vi "Update Task Infos.vi"(8 "error in (no error)":errorcluster, 10 "Task":i32, 11 "Task Setting Editor in":refnum<class "Task Setting Editor.lvclass">) -> (0 "error out":errorcluster, 3 "Task Setting Editor out":refnum<class "Task Setting Editor.lvclass">)   [LabVIEW 2017, in "Task Setting Editor.lvlib" / "Task Setting Editor.lvclass"]
uses:
  Task Setting Editor.lvclass
  Task Setting Editor.lvclass/Task Setting Editor.ctl
  Classes/Task Interface/Task/Task.lvclass/Task.ctl
  Classes/Task Interface/Task/Get Name.vi
  Classes/Task Interface/Task/Get Target.vi
  Classes/Task Interface/Task/Read BuildSpec Type.vi
  Classes/Task Interface/Task/Get BuildSpec Name.vi
  Classes/Task Interface/Task/Get ProjectPath.vi
  Classes/Task Interface/Task/Read Worker.vi
  Classes/Task Interface/Task/Read Display Name.vi
  Classes/Task Interface/Task/Get Status String.vi
  Classes/Task Interface/Task/Get ProjectName.vi
  Classes/Task Interface/Task/Task.lvclass
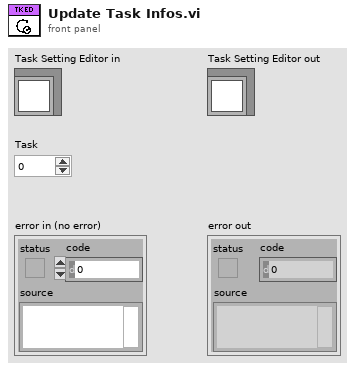
[diagram p1: front panel]
types:
  T1 = cluster{"Display Name":refnum<vi>, "Worker":refnum<vi>}
  T2 = cluster{"Name":refnum<vi>, "ProjectName":refnum<vi>, "Target":refnum<vi>, "BuildSpec Type":refnum<vi>, "BuildSpec Name":refnum<vi>, "ProjectPath":refnum<vi>, "Status string":refnum<vi>}
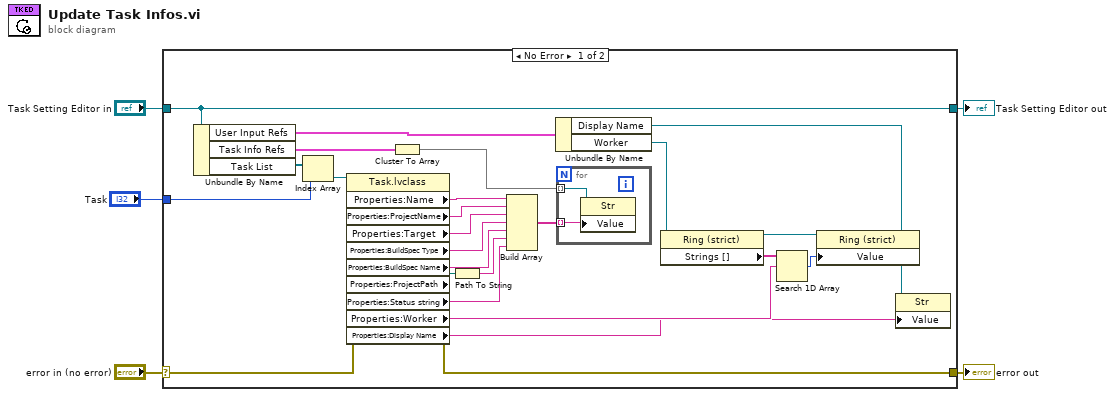
[diagram p0: block diagram]
diagram:
  n1 = case shown="No Error" "error in (no error)" {
    selector: "error in (no error)" -> [w27 w34]
    tunnel: [w26 w34] -> w4
    tunnel: [w30 w33] -> w2
    tunnel: "Task Setting Editor in" -> [w30 w33]
    tunnel: "Task" -> [w28 _]
    frame No Error {
      n2 = Unbundle By Name(w30) -> ("User Input Refs"=w23:T1, "Task Info Refs"=w20:T2, "Task List"=w29:refnum<class "Task.lvclass">[])
      n3 = Index Array(array=w29, index=w28) -> (element=w15:refnum<class "Task.lvclass">)
      n4 = property class="Task.lvclass"(reference=w15, error in=w27) -> (error out=w26:errorcluster, "Properties:Name"=w14:string, "Properties:ProjectName"=w13:string, "Properties:Target"=w12:string, "Properties:BuildSpec Type"=w11:string, "Properties:BuildSpec Name"=w10:string, "Properties:ProjectPath"=w9:path, "Properties:Status string"=w8:string, "Properties:Worker"=w7:string, "Properties:Display Name"=w6:string)  [unwired: 1 out]
      n5 = Cluster To Array(cluster=w20) -> (array=w25:refnum<vi>[])
      n6 = Path To String(path=w9) -> (string=w19:string)
      n7 = Build Array(w14, w13, w12, w11, w10, w19, w8) -> (w24:string[])
      n8 = Unbundle By Name(w23) -> ("Display Name"=w21:refnum<vi>, "Worker"=w22:refnum<vi>)
      n9 = for {
        tunnel: w25 -> [w32] mode=indexing
        tunnel: w24 -> [w31] mode=indexing
        n10 = property class="Str"(reference=w32, "Value"=w31) -> ()  [unwired: 1 in, 2 out]
      }
      n11 = property class="Ring (strict)"(reference=w22) -> (reference out=w17:refnum<vi>, "Strings []"=w18:string[])  [unwired: 1 in, 1 out]
      n12 = Search 1D Array(1D array=w18, element=w7) -> (index of element=w16:i32)  [unwired: 1 in]
      n13 = property class="Ring (strict)"(reference=w17, "Value"=w16) -> ()  [unwired: 1 in, 2 out]
      n14 = property class="Str"(reference=w21, "Value"=w6) -> ()  [unwired: 1 in, 2 out]
    }
    frame Error {
    }
  }
  "error out" <- w4
  "Task Setting Editor out" <- w2
